vi "Interpolate.vi"(10 "X":dbl[](array[numeric]), 11 "Points interpolation":u32) -> (3 "Array":dbl[](array[numeric]))   [LabVIEW 2012]
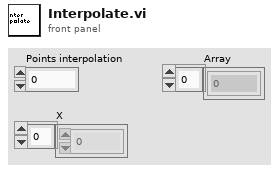
[diagram p1: front panel]
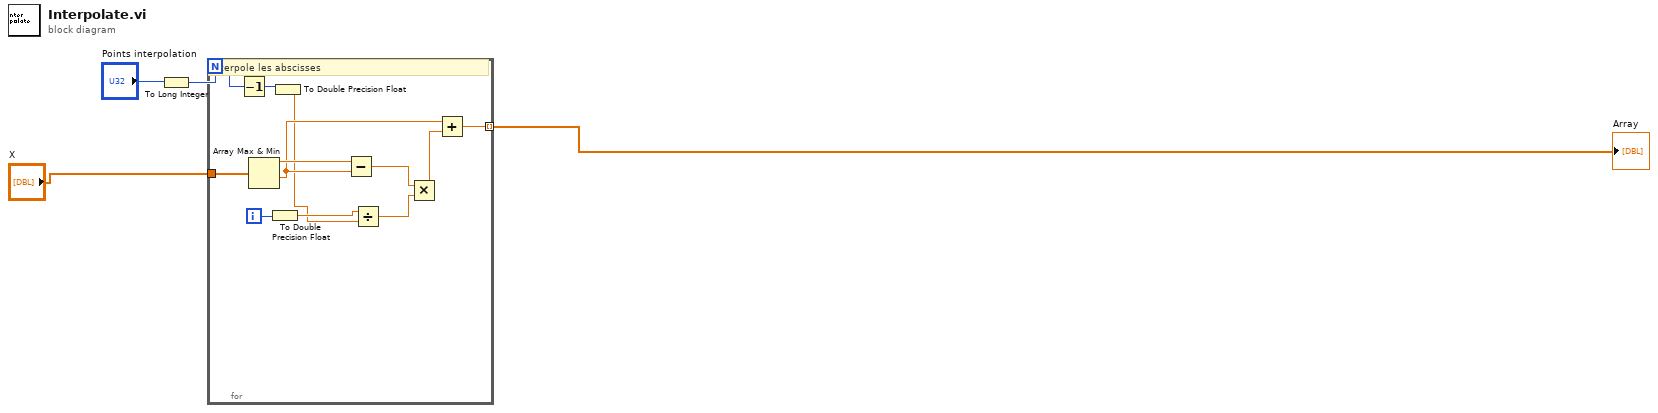
[diagram p0: block diagram]
diagram:
  n1 = To Long Integer(number="Points interpolation") -> (32bit integer=w2:i32)
  n2 = for {
    N: w2 -> [w16]
    tunnel: "X" -> [w15]
    tunnel: [w9] -> w4 mode=indexing
    i -> [w8]
    # "Interpole les abscisses"
    n3 = Decrement(x=w16) -> (x-1=w6:i32)
    n4 = Array Max & Min(array=w15) -> (max value=w12:dbl, min value=w10:dbl)  [unwired: 2 out]
    n5 = To Double Precision Float(number=w8) -> (double precision float=w7:dbl)
    n6 = To Double Precision Float(number=w6) -> (double precision float=w5:dbl)
    n7 = Subtract(x=w12, y=w10) -> (x-y=w14:dbl)
    n8 = Divide(x=w7, y=w5) -> (x/y=w13:dbl)
    n9 = Multiply(x=w14, y=w13) -> (x*y=w11:dbl)
    n10 = Add(x=w10, y=w11) -> (x+y=w9:dbl)
  }
  "Array" <- w4
